vi "GUI_148_AmplifierCams.vi"() -> ()   [LabVIEW 2013]
uses:
  Shared/GUI_Template/GUI_master/tcp_new_data_event.ctl
  Shared/GUI_Template/GUI_master/tcp new data cluster.ctl
  General GUIs/Device GUIs/GUI_Cameras/Controls/Crosshair type def.ctl
  <userlib>/_OpenG.lib/array/array.llb/Filter 1D Array with Scalar (String)__ogtk.vi
panel:
  in  "Analysis::10":bool
  out "MeanCounts::10":dbl caption="updatting?" min=0.0 max=999999999.0 format="%_4g"
  in  "Analysis::9":bool
  out "MeanCounts::9":dbl caption="updatting?" min=0.0 max=999999999.0 format="%_4g"
  in  "Analysis::8":bool
  out "MeanCounts::8":dbl caption="updatting?" min=0.0 max=999999999.0 format="%_4g"
  in  "Analysis::7":bool
  out "MeanCounts::7":dbl caption="updatting?" min=0.0 max=999999999.0 format="%_4g"
  in  "Analysis::6":bool
  out "MeanCounts::6":dbl caption="updatting?" min=0.0 max=999999999.0 format="%_4g"
  in  "Analysis::5":bool
  out "MeanCounts::5":dbl caption="updatting?" min=0.0 max=999999999.0 format="%_4g"
  in  "Analysis::4":bool
  out "MeanCounts::4":dbl caption="updatting?" min=0.0 max=999999999.0 format="%_4g"
  in  "Analysis::3":bool
  out "MeanCounts::3":dbl caption="updatting?" min=0.0 max=999999999.0 format="%_4g"
  in  "Color":u32
  in  "Analysis::2":bool
  out "MeanCounts::2":dbl caption="updatting?" min=0.0 max=999999999.0 format="%_4g"
  in  "triggerdelay::10":dbl=0.001 caption="triggerdelay" min=0.0 max=50000.0 format="%_4p"
  in  "triggerdelay::9":dbl=0.001 caption="triggerdelay" min=0.0 max=0.3 format="%_4p"
  in  "triggerdelay::8":dbl=0.001 caption="triggerdelay" min=16.0 max=50000.0 format="%_4p"
  in  "trigger::10":bool caption="Trigger"
  in  "exposure::10":dbl=0.001 caption="exposure" min=0.0001 max=1.0 format="%_4p"
  in  "trigger::9":bool caption="Trigger"
  in  "exposure::9":dbl=0.001 caption="exposure" min=2e-05 max=1.0 format="%_4p"
  in  "trigger::8":bool caption="Trigger"
  in  "exposure::8":dbl=0.001 caption="exposure" min=0.0001 max=1.0 format="%_4p"
  in  "Target.Y::10":dbl=45.0 caption="y" min=0.0 max=2000.0 format="%#_6f"
  in  "Target.X::10":dbl=47.0 caption="x" min=0.0 max=2000.0 format="%#_6f"
  in  "Target.Y::9":dbl=45.0 caption="y" min=0.0 max=2000.0 format="%#_6f"
  in  "Target.X::9":dbl=47.0 caption="x" min=0.0 max=2000.0 format="%#_6f"
  in  "Target.Y::8":dbl=45.0 caption="y" min=0.0 max=2000.0 format="%#_6f"
  in  "Target.X::8":dbl=47.0 caption="x" min=0.0 max=2000.0 format="%#_6f"
  in  "TargetSize.Y::10":dbl=45.0 caption="y" min=2.0 max=3000.0 format="%#_6f"
  in  "TargetSize.X::10":dbl=47.0 caption="x" min=2.0 max=3000.0 format="%#_6f"
  in  "TargetSize.Y::9":dbl=45.0 caption="y" min=2.0 max=3000.0 format="%#_6f"
  in  "TargetSize.X::9":dbl=47.0 caption="x" min=2.0 max=3000.0 format="%#_6f"
  in  "TargetSize.Y::8":dbl=45.0 caption="y" min=2.0 max=3000.0 format="%#_6f"
  in  "TargetSize.X::8":dbl=47.0 caption="x" min=2.0 max=3000.0 format="%#_6f"
  out "image::10":T1(plugin-control) caption="UC_GAIAMode"
  in  "GUIdevice 10":string="UC_GaiaMode"
  out "image::9":T1(plugin-control) caption="UC_GratingMode"
  in  "GUIdevice 9":string="UC_GratingMode"
  out "image::8":T1(plugin-control) caption="UC_Amp4_IR_output"
  in  "GUIdevice 8":string="UC_Amp4_IR_output"
  in  "TargetSize.Y::7":dbl=45.0 caption="y" min=2.0 max=3000.0 format="%#_6f"
  in  "TargetSize.X::7":dbl=47.0 caption="x" min=2.0 max=3000.0 format="%#_6f"
  in  "TargetSize.Y::6":dbl=45.0 caption="y" min=2.0 max=3000.0 format="%#_6f"
  in  "TargetSize.X::6":dbl=47.0 caption="x" min=2.0 max=3000.0 format="%#_6f"
  in  "TargetSize.Y::5":dbl=45.0 caption="y" min=2.0 max=3000.0 format="%#_6f"
  in  "TargetSize.X::5":dbl=47.0 caption="x" min=2.0 max=3000.0 format="%#_6f"
  in  "TargetSize.Y::4":dbl=45.0 caption="y" min=2.0 max=3000.0 format="%#_6f"
  in  "TargetSize.X::4":dbl=47.0 caption="x" min=2.0 max=3000.0 format="%#_6f"
  in  "TargetSize.Y::3":dbl=163.0 caption="y" min=2.0 max=3000.0 format="%#_6f"
  in  "TargetSize.X::3":dbl=152.0 caption="x" min=2.0 max=3000.0 format="%#_6f"
  in  "TargetSize.Y::2":dbl=74.0 caption="y" min=2.0 max=3000.0 format="%#_6f"
  in  "TargetSize.X::2":dbl=75.0 caption="x" min=2.0 max=3000.0 format="%#_6f"
  in  "active cams":string
  out "CCDs":string[](array[string])
  out "Cameras":T2
  in  "Target.Y::7":dbl=45.0 caption="y" min=0.0 max=2000.0 format="%#_6f"
  in  "Target.X::7":dbl=47.0 caption="x" min=0.0 max=2000.0 format="%#_6f"
  in  "Target.Y::6":dbl=45.0 caption="y" min=0.0 max=2000.0 format="%#_6f"
  in  "Target.X::6":dbl=47.0 caption="x" min=0.0 max=2000.0 format="%#_6f"
  in  "Target.Y::5":dbl=45.0 caption="y" min=0.0 max=2000.0 format="%#_6f"
  in  "Target.X::5":dbl=47.0 caption="x" min=0.0 max=2000.0 format="%#_6f"
  in  "Target.Y::4":dbl=45.0 caption="y" min=0.0 max=2000.0 format="%#_6f"
  in  "Target.X::4":dbl=47.0 caption="x" min=0.0 max=2000.0 format="%#_6f"
  in  "Target.Y::3":dbl=163.0 caption="y" min=0.0 max=2000.0 format="%#_6f"
  in  "Target.X::3":dbl=152.0 caption="x" min=0.0 max=2000.0 format="%#_6f"
  in  "Target.Y::2":dbl=74.0 caption="y" min=0.0 max=2000.0 format="%#_6f"
  in  "Target.X::2":dbl=75.0 caption="x" min=0.0 max=2000.0 format="%#_6f"
  out "error out":errorcluster
  out "image::7":T1(plugin-control) caption="UC_Amp4Depletion_South"
  in  "triggerdelay::7":dbl=0.001 caption="triggerdelay" min=10.0 max=50000.0 format="%_4p"
  in  "triggerdelay::6":dbl=0.001 caption="triggerdelay" min=20.0 max=50000.0 format="%_4p"
  in  "triggerdelay::5":dbl=0.001 caption="triggerdelay" min=10.0 max=50000.0 format="%_4p"
  in  "triggerdelay::4":dbl=0.001 caption="triggerdelay" min=20.0 max=50000.0 format="%_4p"
  in  "triggerdelay::3":dbl=0.001 caption="triggerdelay" min=20.0 max=50000.0 format="%_4p"
  in  "triggerdelay::2":dbl=0.001 caption="triggerdelay" min=0.0 max=50000.0 format="%_4p"
  in  "trigger::7":bool caption="Trigger"
  in  "exposure::7":dbl=0.001 caption="exposure" min=0.0001 max=1.0 format="%_4p"
  in  "GUIdevice 7":string="UC_Amp4Depletion_South"
  in  "trigger::6":bool caption="Trigger"
  in  "exposure::6":dbl=0.001 caption="exposure" min=0.0001 max=1.0 format="%_4p"
  out "image::6":T1(plugin-control) caption="UC_Amp3Depletion_South"
  in  "GUIdevice 6":string="UC_Amp3Depletion_South"
  in  "trigger::5":bool caption="Trigger"
  in  "exposure::5":dbl=0.001 caption="exposure" min=0.0001 max=1.0 format="%_4p"
  out "image::5":T1(plugin-control) caption="UC_Amp2Depletion_South"
  in  "GUIdevice 5":string="UC_Amp2Depletion_South"
  in  "trigger::4":bool caption="Trigger"
  in  "exposure::4":dbl=0.001 caption="exposure" min=0.0001 max=1.0 format="%_4p"
  out "image::4":T1(plugin-control) caption="UC_Amp4_IR_Input"
  in  "GUIdevice 4":string="UC_Amp4_IR_input"
  in  "trigger::3":bool caption="Trigger"
  in  "exposure::3":dbl=0.001 caption="exposure" min=0.0001 max=1.0 format="%_4p"
  out "image::3":T1(plugin-control) caption="UC_Amp3_IR_Input"
  in  "GUIdevice 3":string="UC_Amp3_IR_input"
  in  "trigger::2":bool caption="Trigger"
  in  "exposure::2":dbl=0.001 caption="exposure" min=0.0001 max=1.0 format="%_4p"
  out "image::2":T1(plugin-control) caption="UC_Amp2_IR_input"
  in  "GUIdevice 2":string="UC_Amp2_IR_input"
  out "tcp data event":T3
  in  "Select device":string(combo)="FrogHPD"
  in  "stop":bool
  in  "GUIdevice 1":string="HPD_CCD"
  # "XHair location"
  # "XHair size"
  # "XHair location"
  # "XHair size"
  # "XHair location"
  # "XHair size"
  # "XHair location"
  # "XHair size"
  # "XHair location"
  # "XHair size"
  # "XHair location"
  # "XHair size"
  # "XHair location"
  # "XHair size"
  # "XHair location"
  # "XHair size"
  # "XHair location"
  # "XHair size"
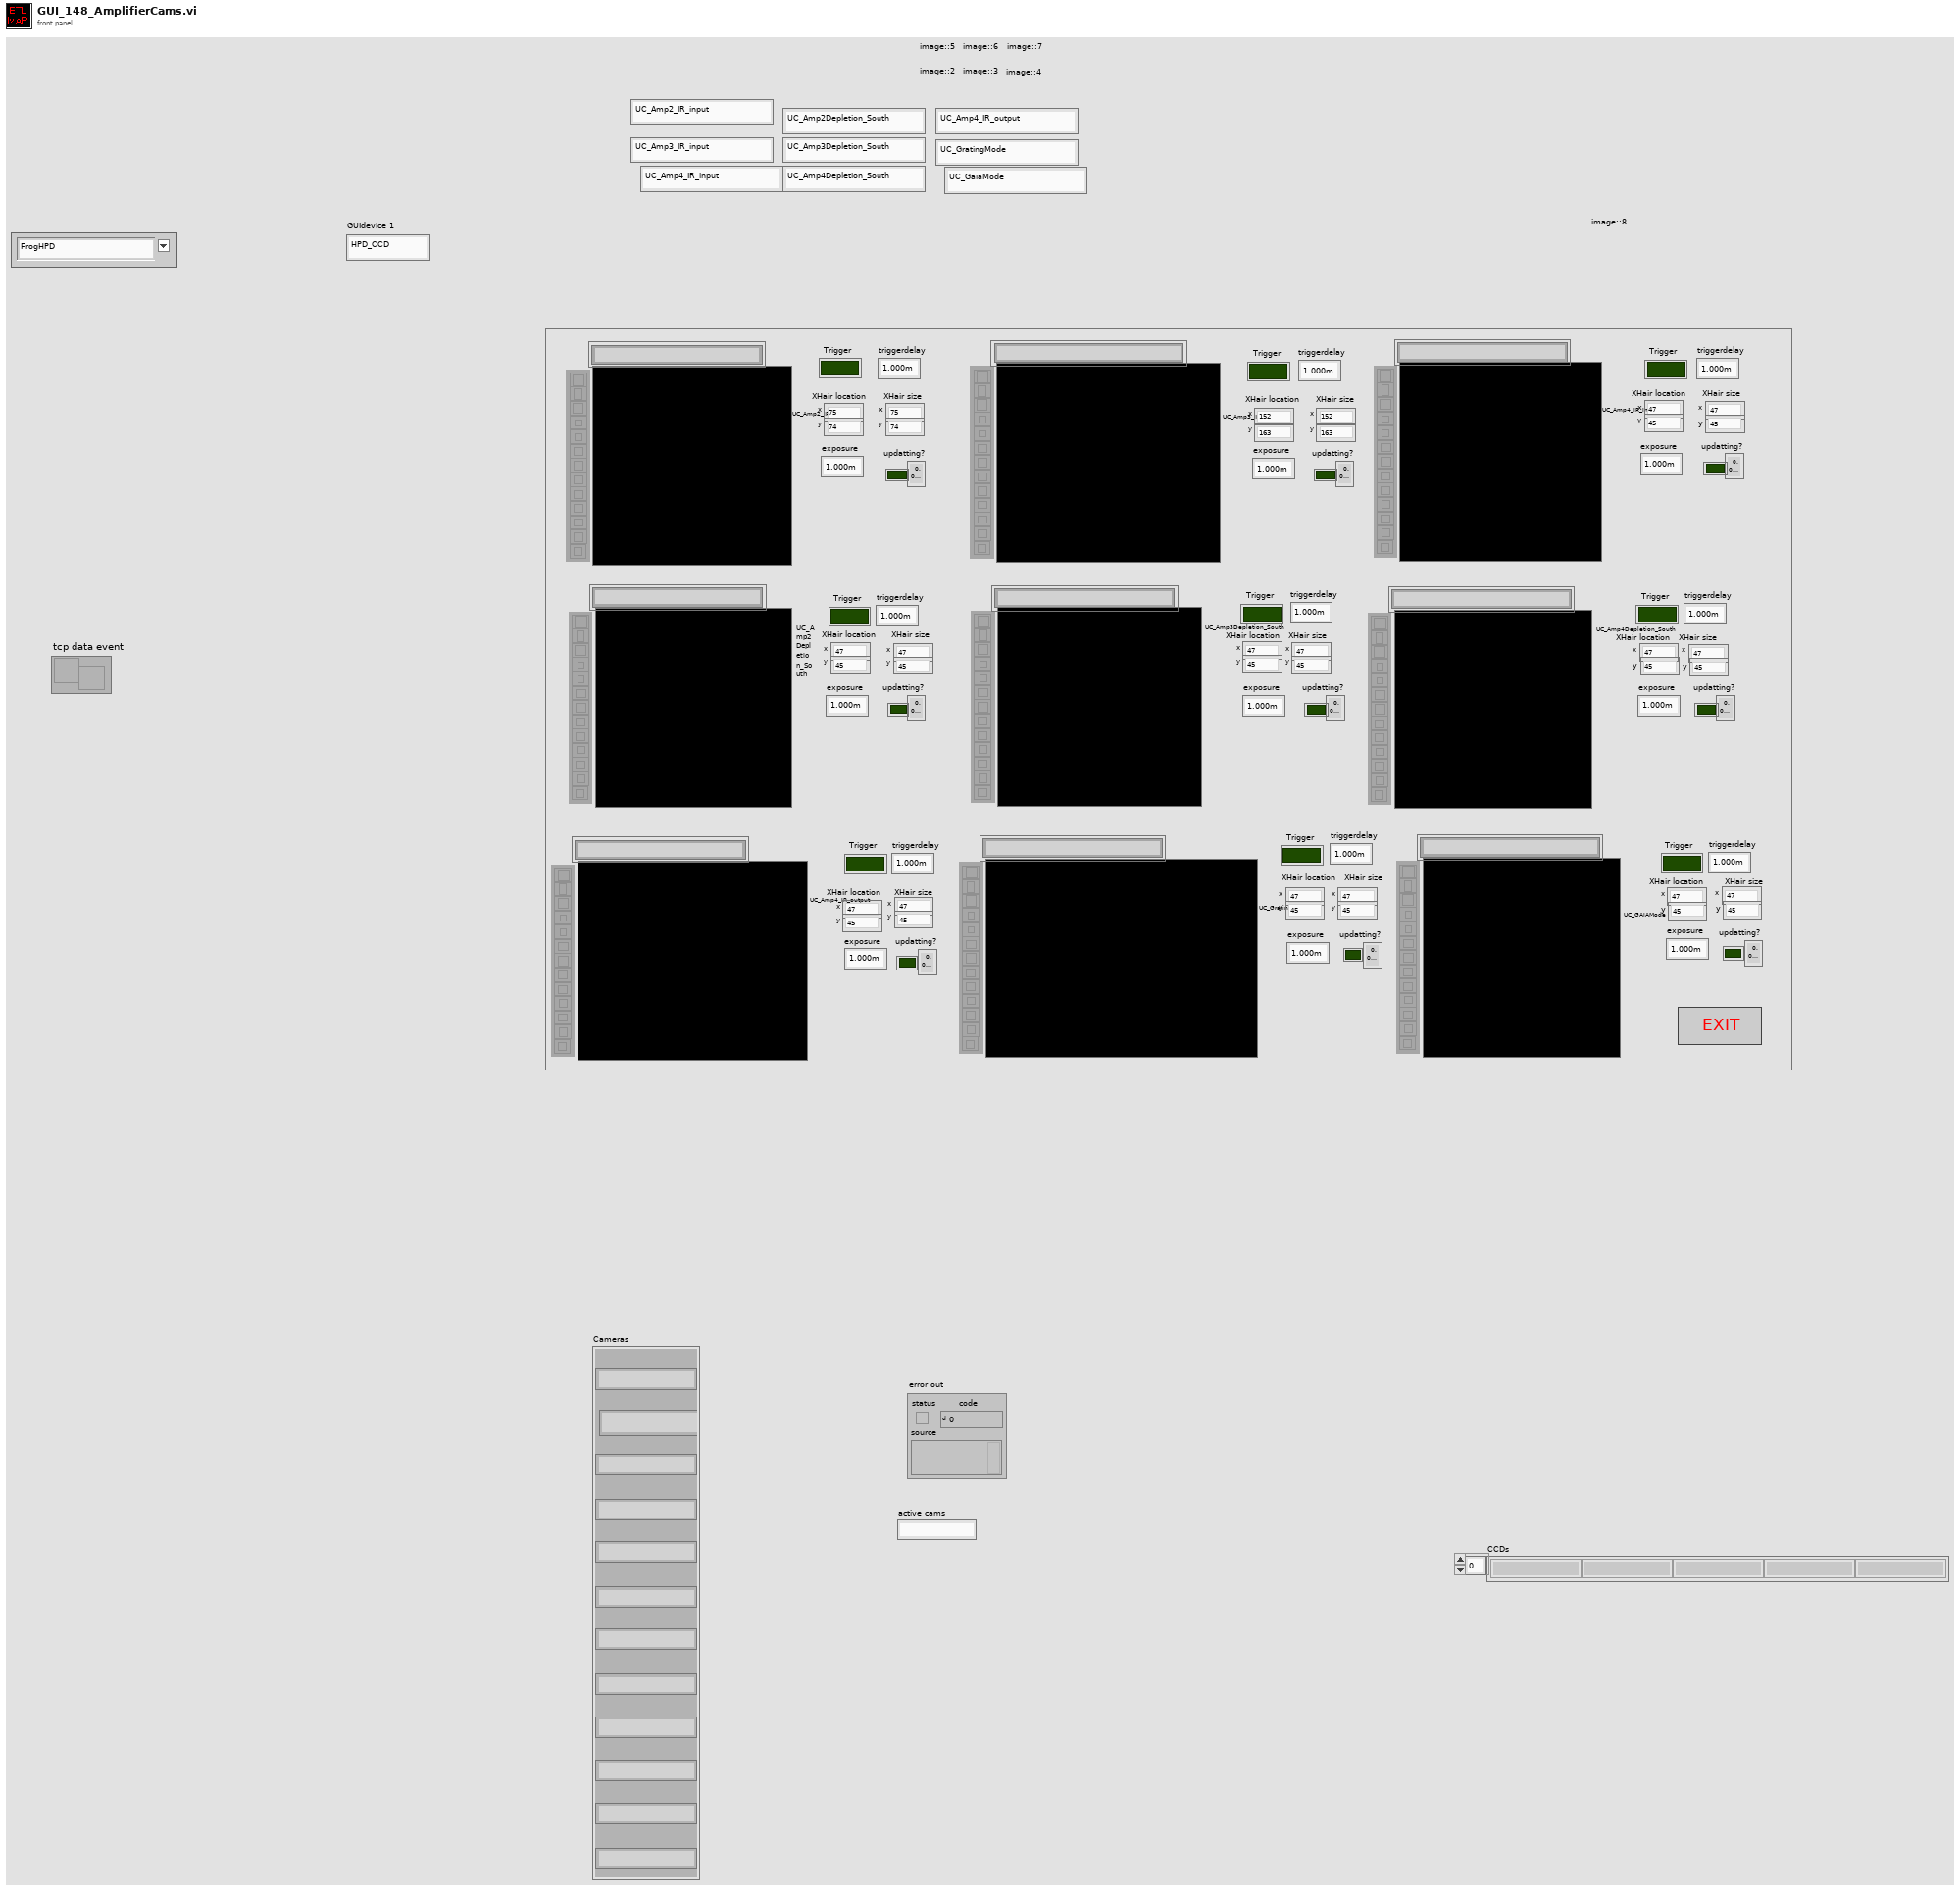
[diagram p1: front panel]
types:
  T1 = typedef "IMAQ Image.ctl" = refnum<image>
  T2 = cluster{"[0]":string, "[1]":string, "[2]":string, "[3]":string, "[4]":string, "[5]":string, "[6]":string, "[7]":string, "[8]":string, "[8] 2":string, "[8] 3":string, "[8] 4":string}
  T3 = typedef "tcp_new_data_event.ctl" = refnum<user-event>
  T4 = typedef "Image Type" = u32
  T5 = cluster{"Target.X::8":refnum<vi>, "Target.Y::8":refnum<vi>}
  T6 = cluster{"Target.X::9":refnum<vi>, "Target.Y::9":refnum<vi>}
  T7 = cluster{"Target.X::10":refnum<vi>, "Target.Y::10":refnum<vi>}
  T8 = cluster{"Target.X::2":refnum<vi>, "Target.Y::2":refnum<vi>}
  T9 = cluster{"Target.X::3":refnum<vi>, "Target.Y::3":refnum<vi>}
  T10 = cluster{"Target.X::4":refnum<vi>, "Target.Y::4":refnum<vi>}
  T11 = cluster{"Target.X::5":refnum<vi>, "Target.Y::5":refnum<vi>}
  T12 = cluster{"Target.X::6":refnum<vi>, "Target.Y::6":refnum<vi>}
  T13 = cluster{"Target.X::7":refnum<vi>, "Target.Y::7":refnum<vi>}
  T14 = cluster{"TargetSize.X::4":refnum<vi>, "TargetSize.Y::4":refnum<vi>}
  T15 = cluster{"TargetSize.X::5":refnum<vi>, "TargetSize.Y::5":refnum<vi>}
  T16 = cluster{"TargetSize.X::6":refnum<vi>, "TargetSize.Y::6":refnum<vi>}
  T17 = cluster{"TargetSize.X::7":refnum<vi>, "TargetSize.Y::7":refnum<vi>}
  T18 = cluster{"TargetSize.X::8":refnum<vi>, "TargetSize.Y::8":refnum<vi>}
  T19 = cluster{"TargetSize.X::9":refnum<vi>, "TargetSize.Y::9":refnum<vi>}
  T20 = cluster{"TargetSize.X::10":refnum<vi>, "TargetSize.Y::10":refnum<vi>}
  T21 = cluster{"TargetSize.X::2":refnum<vi>, "TargetSize.Y::2":refnum<vi>}
  T22 = cluster{"TargetSize.X::3":refnum<vi>, "TargetSize.Y::3":refnum<vi>}
  T23 = cluster{"[0]":string, "[1]":string, "[2]":string, "[3]":string, "[4]":string, "[5]":string, "[6]":string, "[7]":string, "[8]":string, "[9]":string, "[10]":string, "[11]":string}
  T24 = cluster{"TargetSize.X::10":refnum<vi>, "TargetSize.Y::10":refnum<vi>}[]
  T25 = cluster{"Target.X::10":refnum<vi>, "Target.Y::10":refnum<vi>}[]
  T26 = typedef "Crosshair type def.ctl" = cluster{"Draw":bool, "Target":cluster{"x":dbl, "y":dbl}, "Size":cluster{"x":dbl, "y":dbl}, "Angle":dbl, "Color":u32, "Thickness":u8, "CrosshairLabel":string}
  T27 = cluster{"Left":i32, "Top":i32, "Right":i32, "Bottom":i32}
  T28 = enum32{"invalid app kind", "Development System", "Run Time System", "Student Edition", "Embedded LabVIEW", "Evaluation", "Custom"}
  T29 = typedef "tcp new data cluster.ctl" = cluster{"EventEnum":enum16{"new data", "connection status update"}, "Device name":string}
  T30 = enum32{"Invalid", "Standard", "Closed", "Hidden", "Minimized", "Maximized"}
  T31 = cluster{"Core":cluster{"Current VI Reference":refnum<vi>, "Close Panel on Exit?":bool}, "Your Boolean data":bool, "active cams":string, "SuperGUI":cluster{"STOP queue":refnum<queue>, "SuperGUI ref":refnum<vi>}}
  T32 = cluster{"STOP queue":refnum<queue>, "SuperGUI ref":refnum<vi>}
  T33 = cluster{"Current VI Reference":refnum<vi>, "Close Panel on Exit?":bool}
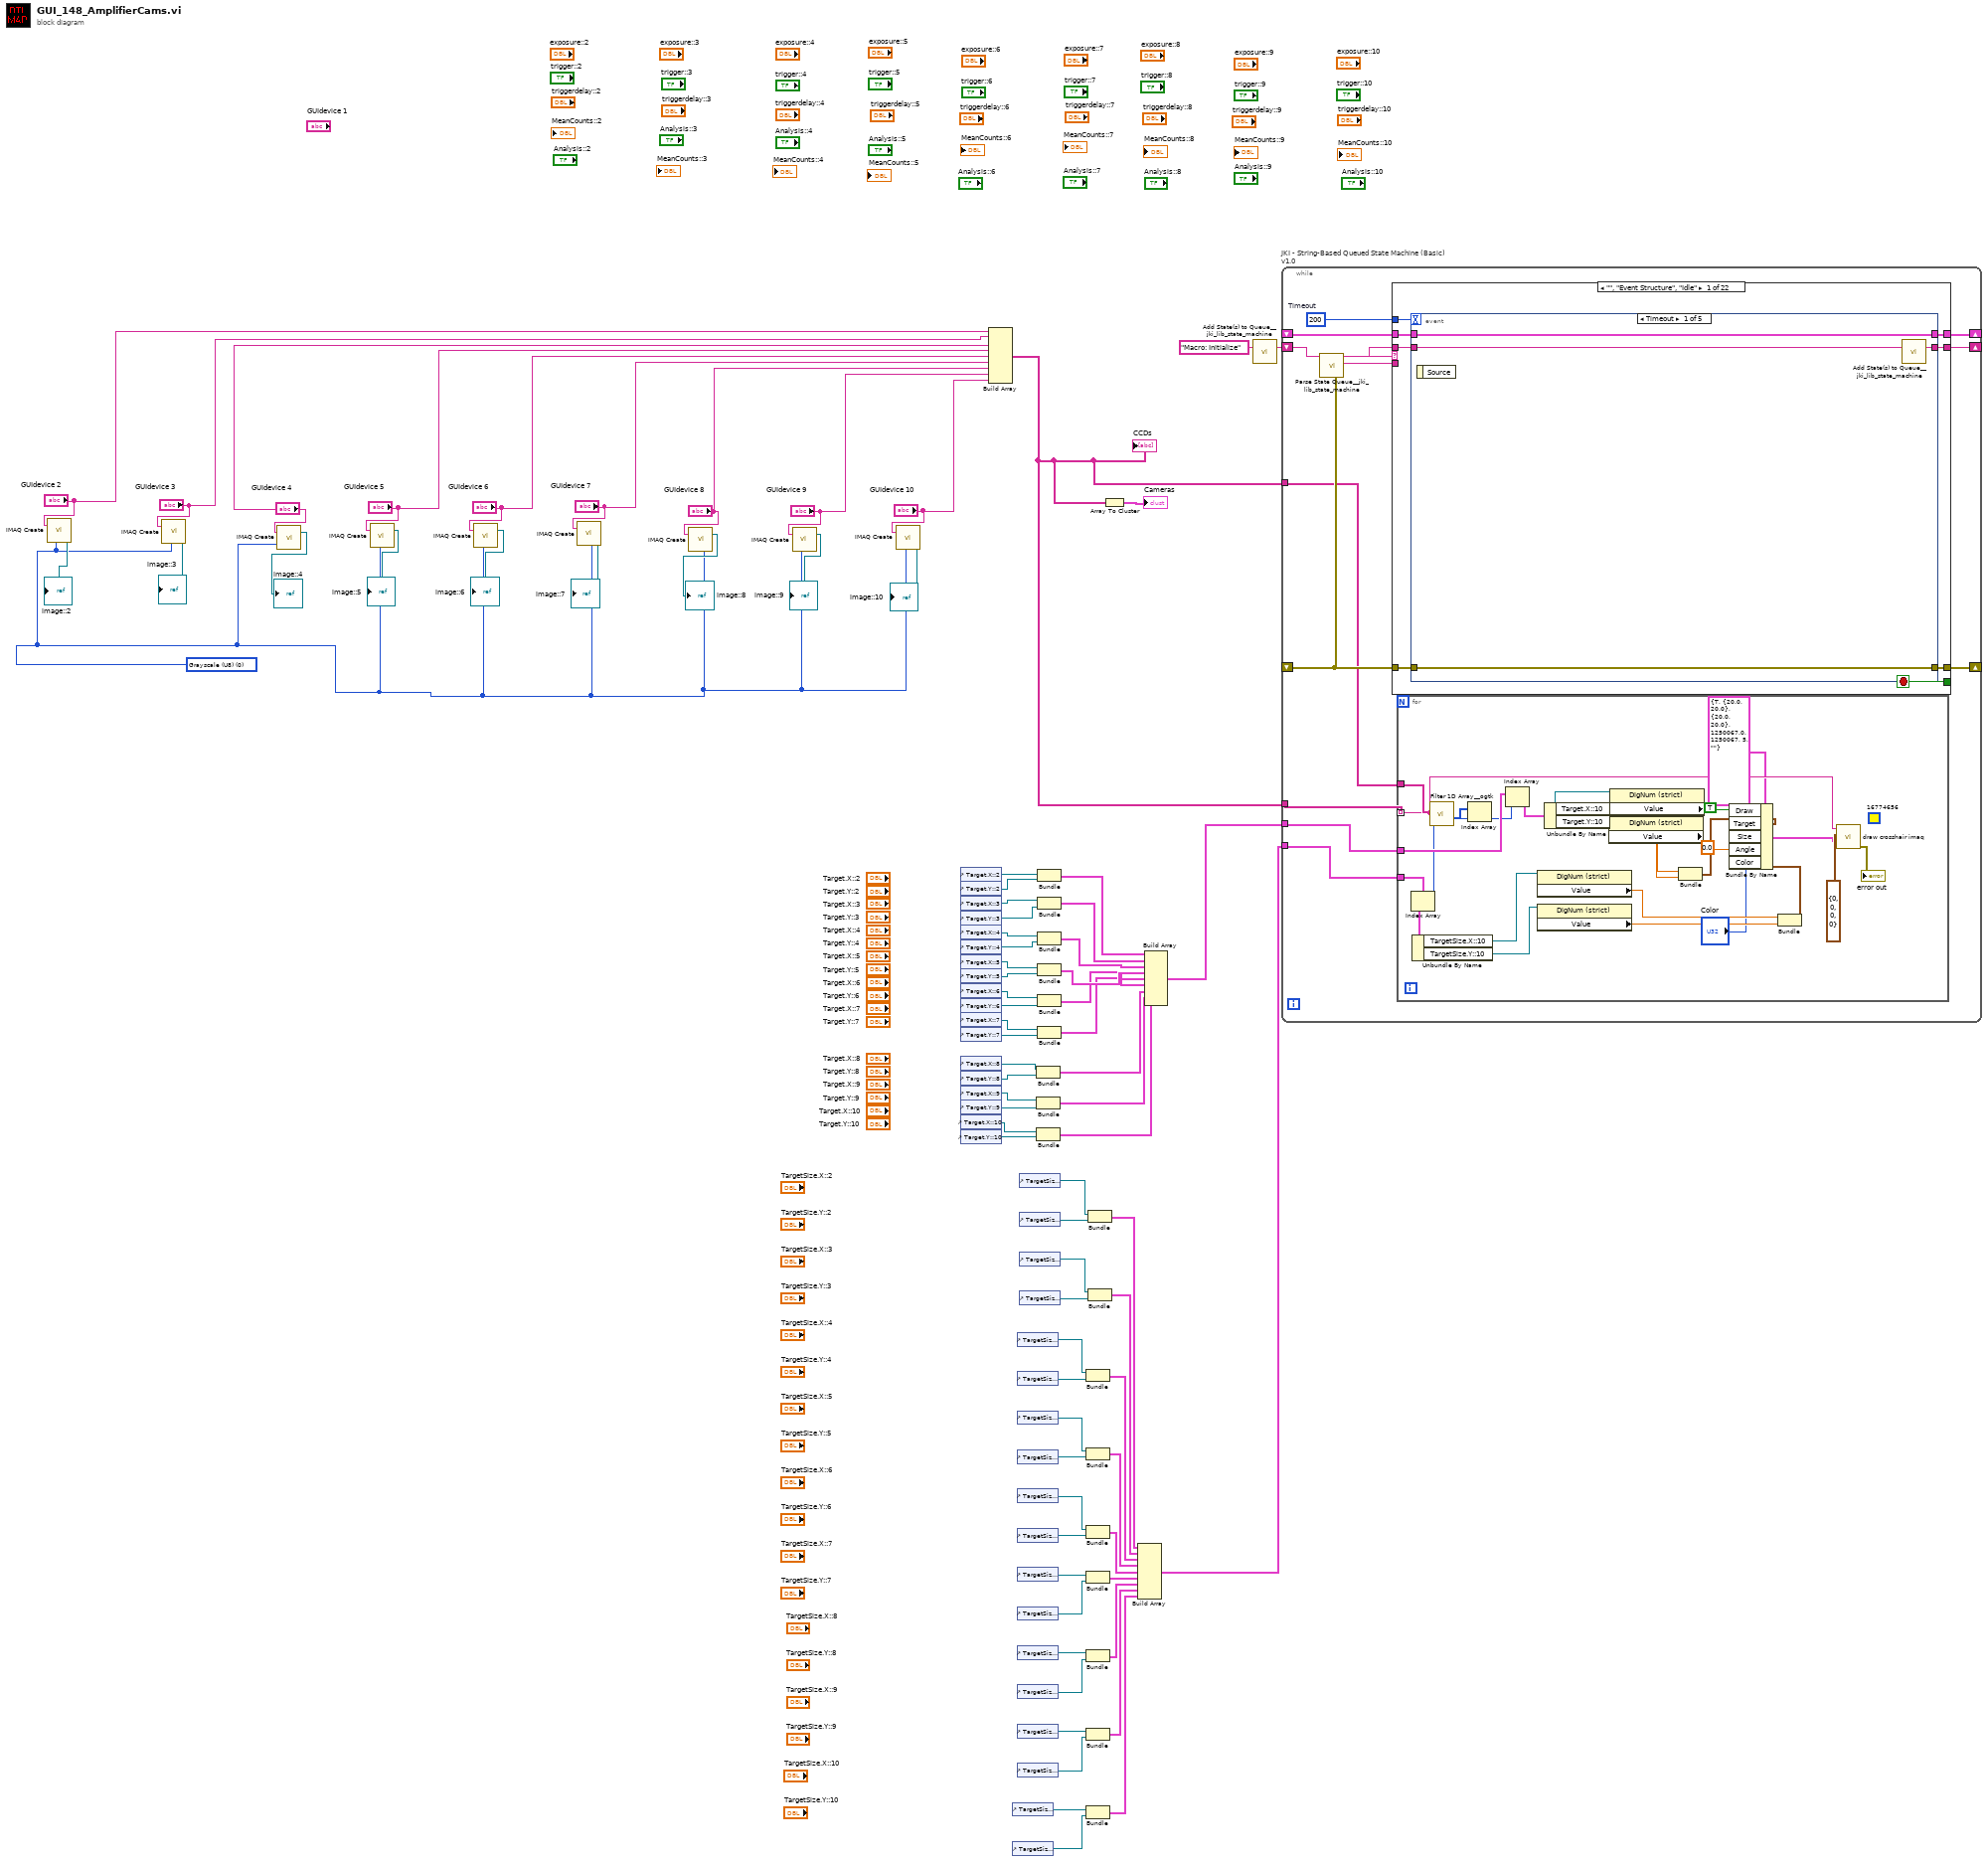
[diagram p0: block diagram]
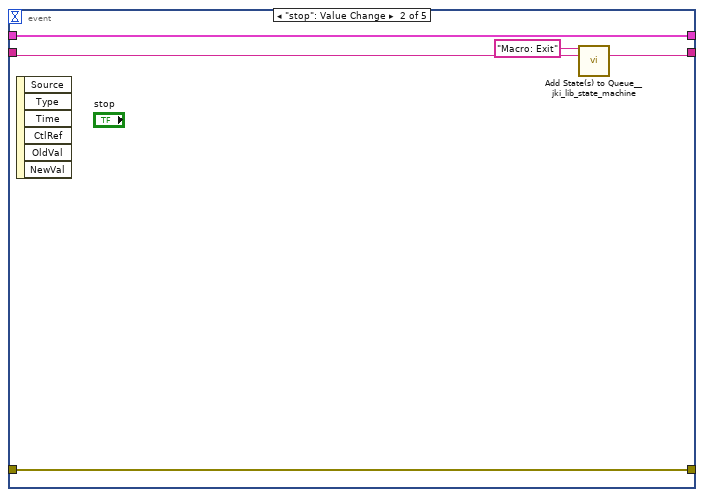
[diagram p2: hidden frame]
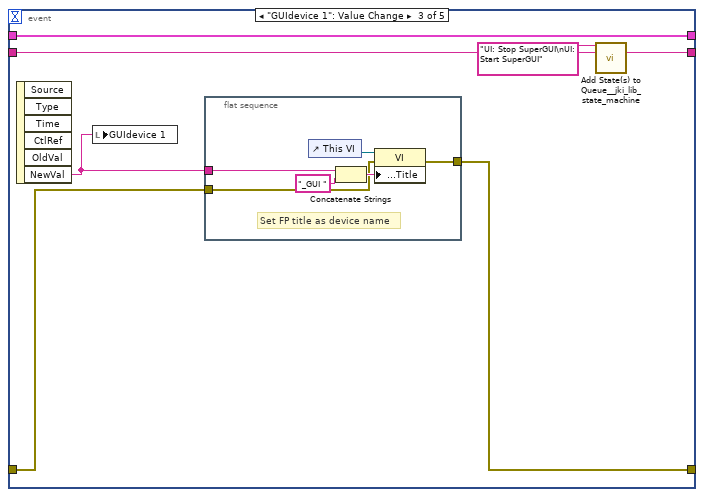
[diagram p3: hidden frame]
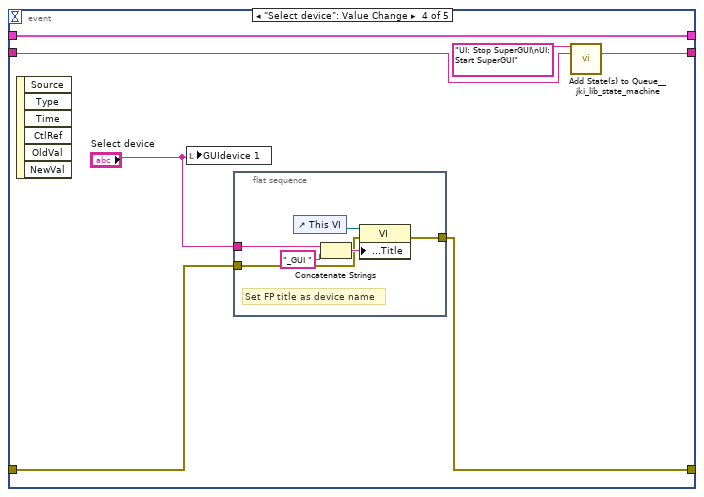
[diagram p4: hidden frame]
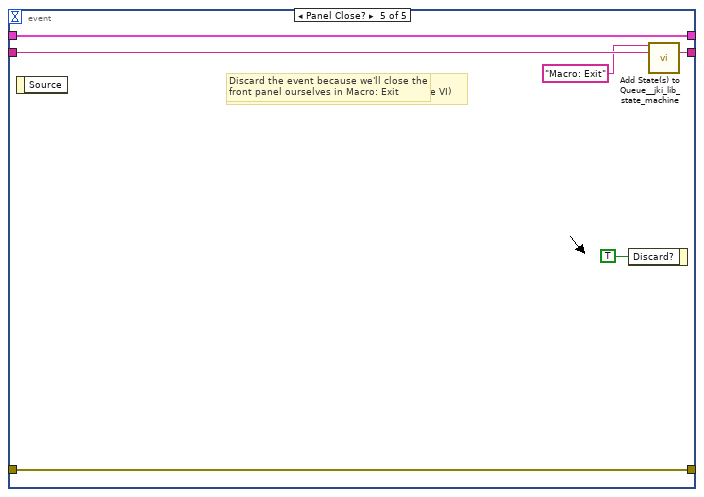
[diagram p5: hidden frame]
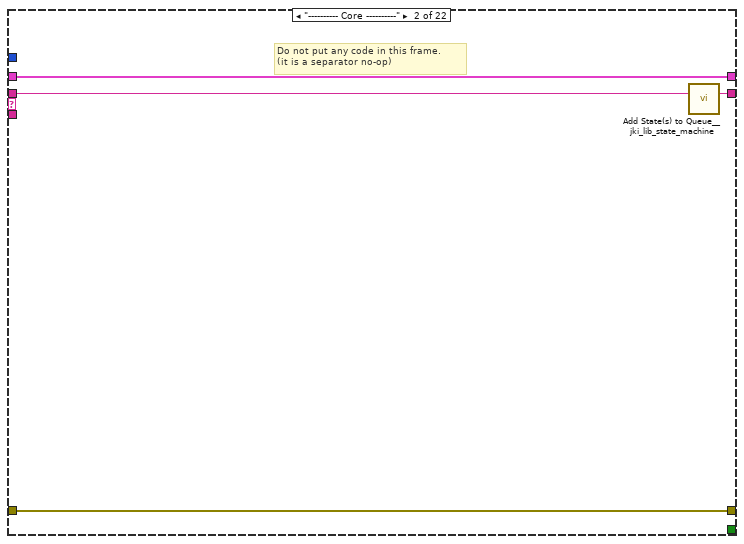
[diagram p6: hidden frame]
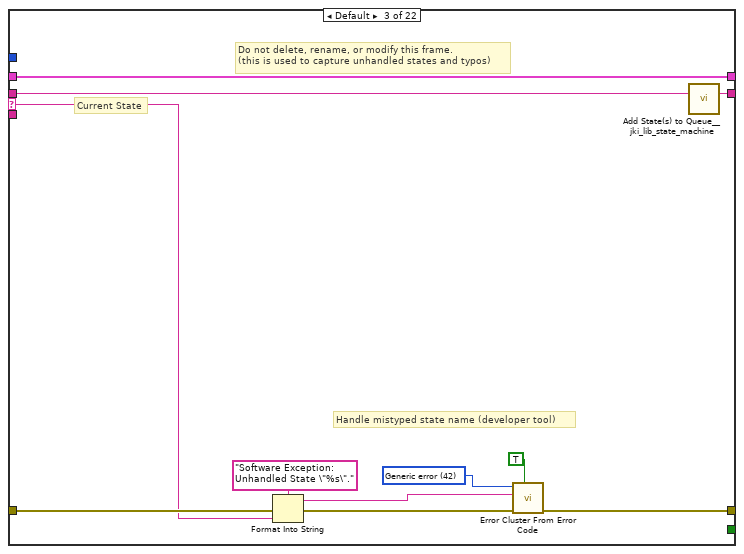
[diagram p7: hidden frame]
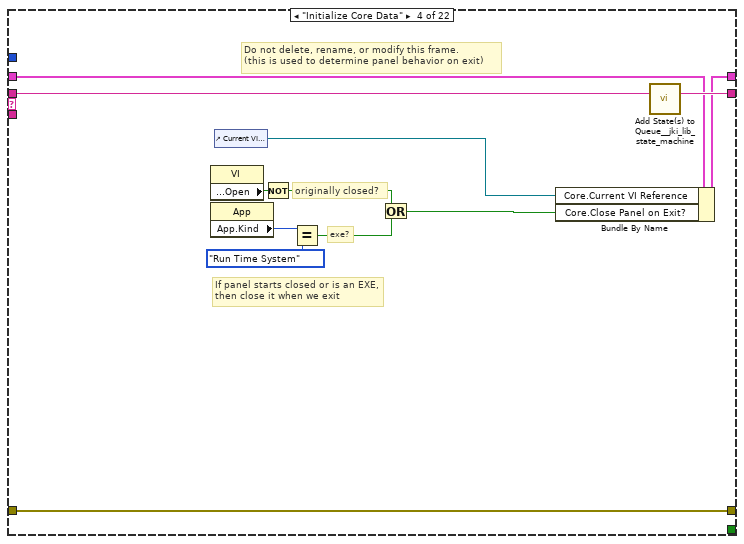
[diagram p8: hidden frame]
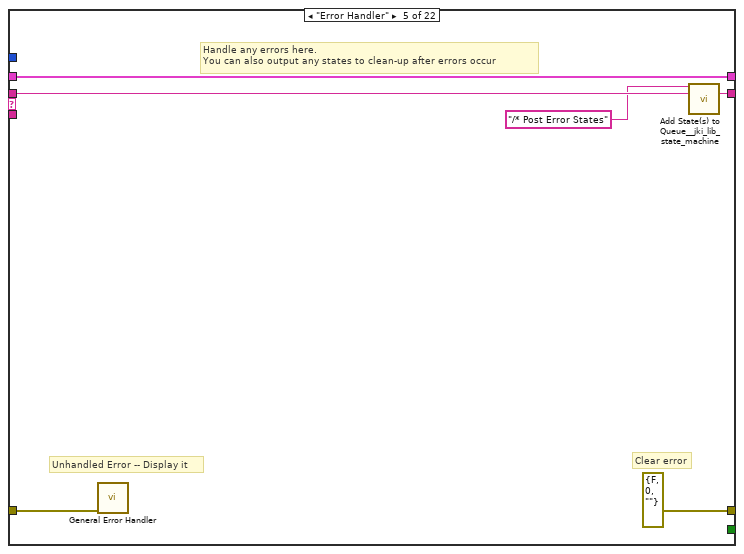
[diagram p9: hidden frame]
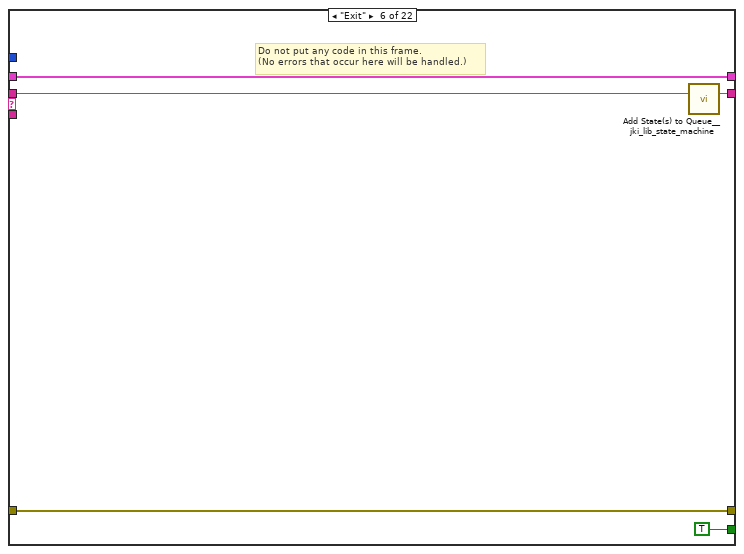
[diagram p10: hidden frame]
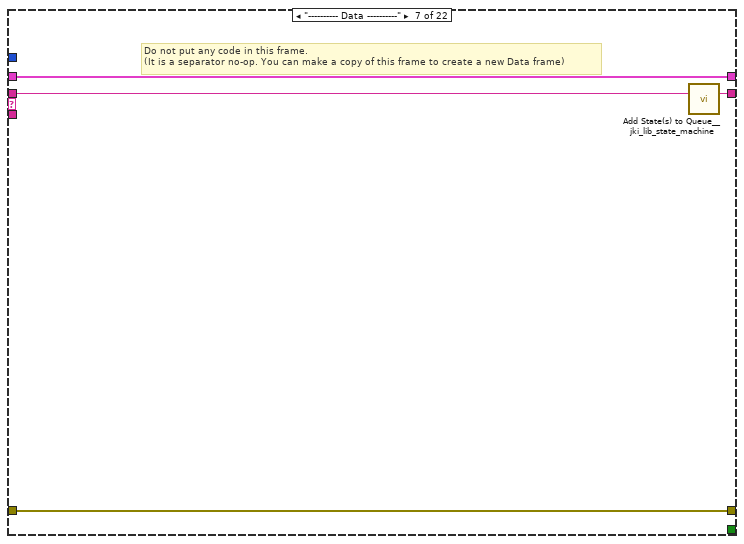
[diagram p11: hidden frame]
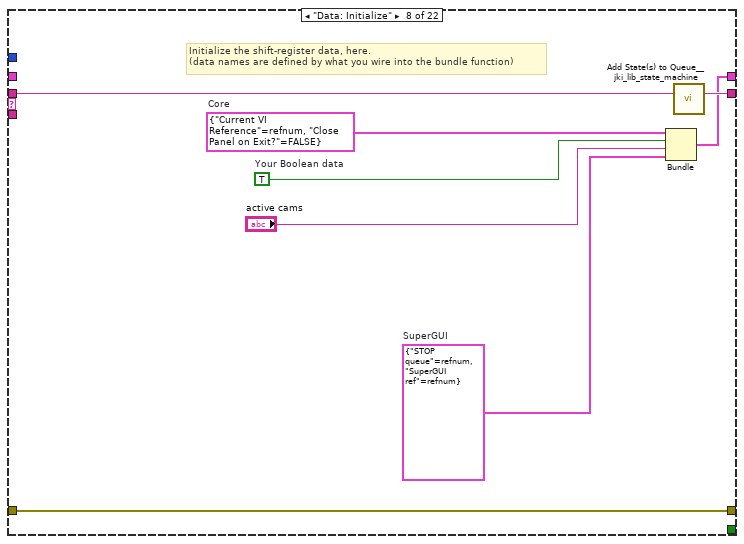
[diagram p12: hidden frame]
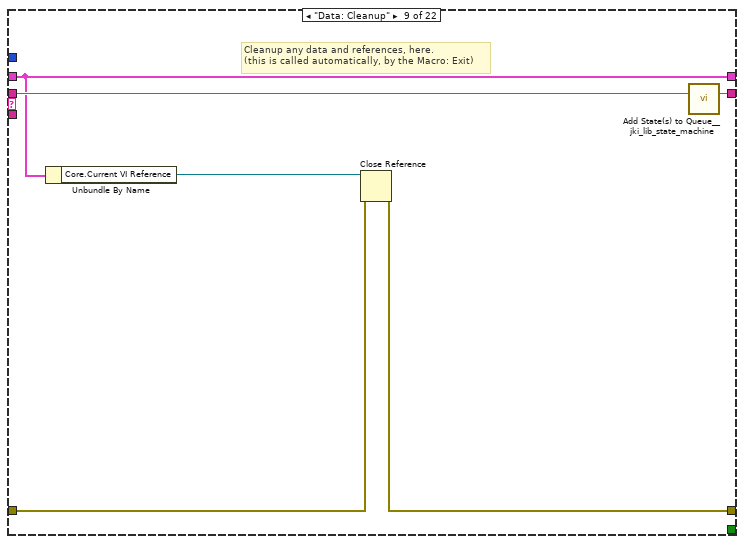
[diagram p13: hidden frame]
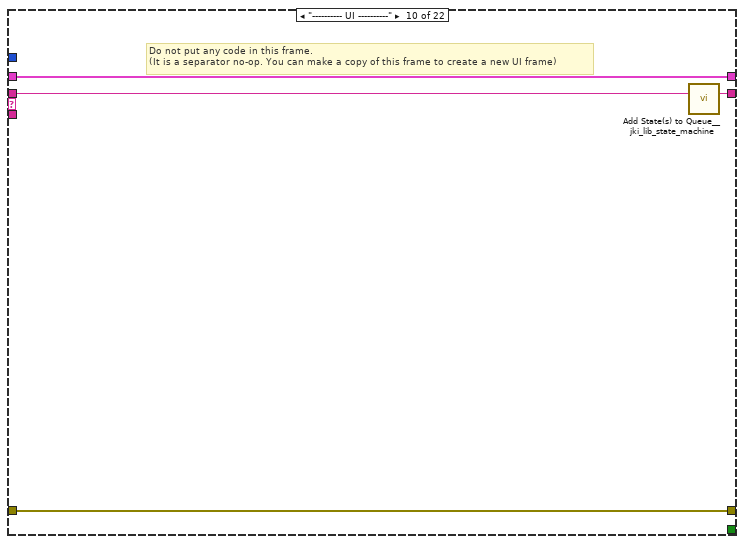
[diagram p14: hidden frame]
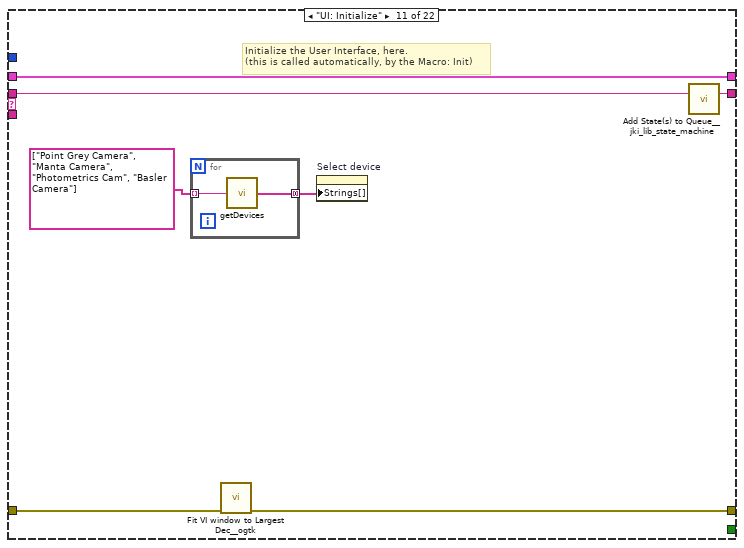
[diagram p15: hidden frame]
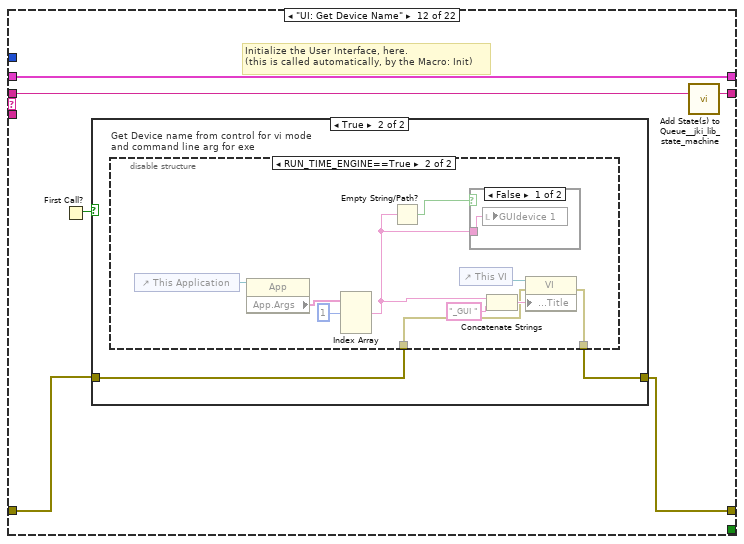
[diagram p16: hidden frame]
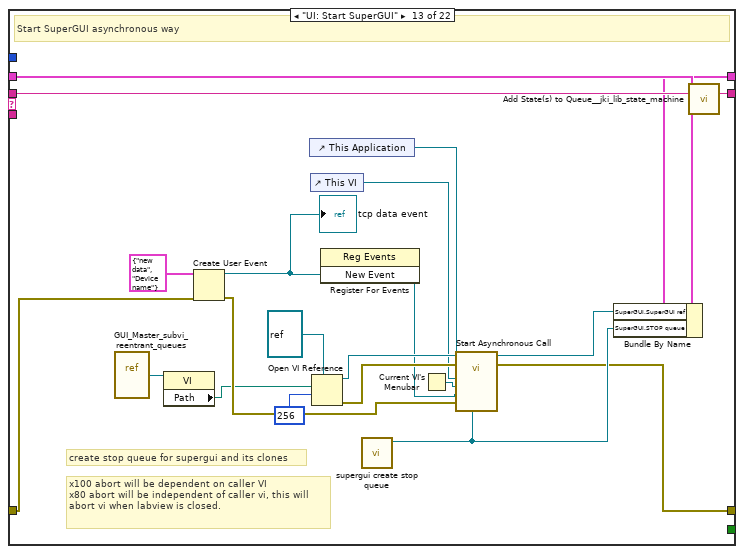
[diagram p20: hidden frame]
diagram:
  w22 = T4 0 items=["Grayscale (U8)", "Grayscale (I16)", "Grayscale (SGL)", "Complex (CSG)", "RGB (U32)", "HSL (U32)", "RGB (U64)", "Grayscale (U16)"] ("Image Type")
  n1 = call "IMAQ Create"("Image Name"="GUIdevice 2", "Image Type"=w22) -> ("New Image"=→"image::2":T1)  [unwired: 3 in, 1 out]
  n2 = call "IMAQ Create"("Image Name"="GUIdevice 3", "Image Type"=w22) -> ("New Image"=→"image::3":T1)  [unwired: 3 in, 1 out]
  n3 = call "IMAQ Create"("Image Name"="GUIdevice 4", "Image Type"=w22) -> ("New Image"=→"image::4":T1)  [unwired: 3 in, 1 out]
  n4 = call "IMAQ Create"("Image Name"="GUIdevice 5", "Image Type"=w22) -> ("New Image"=→"image::5":T1)  [unwired: 3 in, 1 out]
  n5 = call "IMAQ Create"("Image Name"="GUIdevice 6", "Image Type"=w22) -> ("New Image"=→"image::6":T1)  [unwired: 3 in, 1 out]
  n6 = call "IMAQ Create"("Image Name"="GUIdevice 7", "Image Type"=w22) -> ("New Image"=→"image::7":T1)  [unwired: 3 in, 1 out]
  n7 = call "IMAQ Create"("Image Name"="GUIdevice 8", "Image Type"=w22) -> ("New Image"=→"image::8":T1)  [unwired: 3 in, 1 out]
  n8 = call "IMAQ Create"("Image Name"="GUIdevice 9", "Image Type"=w22) -> ("New Image"=→"image::9":T1)  [unwired: 3 in, 1 out]
  n9 = call "IMAQ Create"("Image Name"="GUIdevice 10", "Image Type"=w22) -> ("New Image"=→"image::10":T1)  [unwired: 3 in, 1 out]
  n10 = control-ref of="Target.X::2"() -> (w71:refnum<vi>)
  n11 = control-ref of="Target.Y::2"() -> (w70:refnum<vi>)
  n12 = control-ref of="Target.X::3"() -> (w69:refnum<vi>)
  n13 = control-ref of="Target.Y::3"() -> (w68:refnum<vi>)
  n14 = control-ref of="Target.X::4"() -> (w67:refnum<vi>)
  n15 = control-ref of="Target.Y::4"() -> (w66:refnum<vi>)
  n16 = control-ref of="Target.X::5"() -> (w65:refnum<vi>)
  n17 = control-ref of="Target.Y::5"() -> (w64:refnum<vi>)
  n18 = control-ref of="Target.X::6"() -> (w63:refnum<vi>)
  n19 = control-ref of="Target.Y::6"() -> (w62:refnum<vi>)
  n20 = control-ref of="Target.X::7"() -> (w61:refnum<vi>)
  n21 = control-ref of="Target.Y::7"() -> (w60:refnum<vi>)
  n22 = control-ref of="Target.X::8"() -> (w6:refnum<vi>)
  n23 = control-ref of="Target.Y::8"() -> (w5:refnum<vi>)
  n24 = control-ref of="Target.X::9"() -> (w4:refnum<vi>)
  n25 = control-ref of="Target.Y::9"() -> (w3:refnum<vi>)
  n26 = control-ref of="Target.X::10"() -> (w2:refnum<vi>)
  n27 = control-ref of="Target.Y::10"() -> (w1:refnum<vi>)
  n28 = Build Array("GUIdevice 2", "GUIdevice 3", "GUIdevice 4", "GUIdevice 5", "GUIdevice 6", "GUIdevice 7", "GUIdevice 8", "GUIdevice 9", "GUIdevice 10") -> (w45:string[])
  "CCDs" <- w45
  n29 = control-ref of="TargetSize.X::10"() -> (w11:refnum<vi>)
  n30 = control-ref of="TargetSize.Y::10"() -> (w10:refnum<vi>)
  n31 = control-ref of="TargetSize.X::4"() -> (w40:refnum<vi>)
  n32 = control-ref of="TargetSize.Y::4"() -> (w39:refnum<vi>)
  n33 = control-ref of="TargetSize.X::5"() -> (w38:refnum<vi>)
  n34 = control-ref of="TargetSize.Y::5"() -> (w37:refnum<vi>)
  n35 = control-ref of="TargetSize.X::6"() -> (w36:refnum<vi>)
  n36 = control-ref of="TargetSize.Y::6"() -> (w35:refnum<vi>)
  n37 = control-ref of="TargetSize.X::7"() -> (w34:refnum<vi>)
  n38 = control-ref of="TargetSize.Y::7"() -> (w33:refnum<vi>)
  n39 = control-ref of="TargetSize.X::8"() -> (w15:refnum<vi>)
  n40 = control-ref of="TargetSize.Y::8"() -> (w14:refnum<vi>)
  n41 = control-ref of="TargetSize.X::9"() -> (w13:refnum<vi>)
  n42 = control-ref of="TargetSize.Y::9"() -> (w12:refnum<vi>)
  n43 = control-ref of="TargetSize.X::2"() -> (w44:refnum<vi>)
  n44 = control-ref of="TargetSize.Y::2"() -> (w43:refnum<vi>)
  n45 = control-ref of="TargetSize.X::3"() -> (w42:refnum<vi>)
  n46 = control-ref of="TargetSize.Y::3"() -> (w41:refnum<vi>)
  n47 = Bundle("Target.X::8"=w6, "Target.Y::8"=w5) -> (w18:T5)  [unwired: 1 in]
  n48 = Bundle("Target.X::9"=w4, "Target.Y::9"=w3) -> (w17:T6)  [unwired: 1 in]
  n49 = Bundle("Target.X::10"=w2, "Target.Y::10"=w1) -> (w16:T7)  [unwired: 1 in]
  n50 = Bundle("Target.X::2"=w71, "Target.Y::2"=w70) -> (w59:T8)  [unwired: 1 in]
  n51 = Bundle("Target.X::3"=w69, "Target.Y::3"=w68) -> (w58:T9)  [unwired: 1 in]
  n52 = Bundle("Target.X::4"=w67, "Target.Y::4"=w66) -> (w54:T10)  [unwired: 1 in]
  n53 = Bundle("Target.X::5"=w65, "Target.Y::5"=w64) -> (w57:T11)  [unwired: 1 in]
  n54 = Bundle("Target.X::6"=w63, "Target.Y::6"=w62) -> (w56:T12)  [unwired: 1 in]
  n55 = Bundle("Target.X::7"=w61, "Target.Y::7"=w60) -> (w55:T13)  [unwired: 1 in]
  n56 = Bundle("TargetSize.X::4"=w40, "TargetSize.Y::4"=w39) -> (w27:T14)  [unwired: 1 in]
  n57 = Bundle("TargetSize.X::5"=w38, "TargetSize.Y::5"=w37) -> (w30:T15)  [unwired: 1 in]
  n58 = Bundle("TargetSize.X::6"=w36, "TargetSize.Y::6"=w35) -> (w29:T16)  [unwired: 1 in]
  n59 = Bundle("TargetSize.X::7"=w34, "TargetSize.Y::7"=w33) -> (w28:T17)  [unwired: 1 in]
  n60 = Bundle("TargetSize.X::8"=w15, "TargetSize.Y::8"=w14) -> (w9:T18)  [unwired: 1 in]
  n61 = Bundle("TargetSize.X::9"=w13, "TargetSize.Y::9"=w12) -> (w8:T19)  [unwired: 1 in]
  n62 = Bundle("TargetSize.X::10"=w11, "TargetSize.Y::10"=w10) -> (w7:T20)  [unwired: 1 in]
  n63 = Bundle("TargetSize.X::2"=w44, "TargetSize.Y::2"=w43) -> (w32:T21)  [unwired: 1 in]
  n64 = Bundle("TargetSize.X::3"=w42, "TargetSize.Y::3"=w41) -> (w31:T22)  [unwired: 1 in]
  n65 = Array To Cluster(array=w45) -> (cluster=→"Cameras":T23)
  n66 = Build Array(w32, w31, w27, w30, w29, w28, w9, w8, w7) -> (w26:T24)
  n67 = Build Array(w59, w58, w54, w57, w56, w55, w18, w17, w16) -> (w53:T25)
  n68 = call <vilib>:"Add State(s) to Queue__jki_lib_state_machine.vi"("State(s) in (\"\")"="Macro: Initialize") -> ("States Out"=w79:string)  [unwired: 14 in]
  n69 = while "JKI - String-Based Queued State Machine (Basic) v1.0" {
    shift-right: [w87] -> _
    shift-left: _ -> [w82]
    shift-right: [w90] -> _
    shift-left: _ -> [w85]
    shift-right: [w89] -> _
    shift-left: w79 -> [w91]
    tunnel: w53 -> [w84]
    tunnel: w45 -> [w83]
    tunnel: w45 -> [w81]
    tunnel: w26 -> [w80]
    stop <- w88 stop-if-true
    w86 = 200  # Timeout
    n70 = call <vilib>:"Parse State Queue__jki_lib_state_machine.vi"("State Queue"=w91, "Error In (no error)"=w85) -> ("Remaining States"=w93:string, "Current State"=w94:string, "Arguments"=w92:string)  [unwired: 11 in]
    n71 = case shown="\"\", \"Event Structure\", \"Idle\"" w94 {
      selector: w94 -> [_ _ w172 _ _ _ _ _ _ _ _ _ _ _ _ _ _ _ _ _ _ _]
      tunnel: w93 -> [w126 w171 w176 w194 w200 w205 w209 w217 w223 w227 w234 w242 w277 w285 w291 w302 w328 w333 w343 w347 w351 w355]
      tunnel: w92 -> [_ _ _ _ _ _ _ _ _ _ _ _ _ _ w286 w296 _ _ _ _ _ _]
      tunnel: w82 -> [w124 w168 w174 w185 w197 w203 w206 _ w218 w224 w232 w240 w268 w280 w289 w298 w325 w330 w340 w344 w348 w352]
      tunnel: [w123 w169 w178 w191 errorcluster {"status"=FALSE, "code"=0, "source"=""} ("error out") w202 w207 w214 w219 w225 w230 w237 w261 w278 w287 w299 w326 w331 w341 w345 w349 w353] -> w90
      tunnel: w85 -> [w122 w169 w177 w191 w196 w202 w207 w214 w220 w225 w231 w238 w262 w279 w288 w300 w326 w331 w341 w345 w349 w353]
      tunnel: [w125 w170 w175 w193 w199 w204 w208 w216 w222 w226 w233 w241 w276 w284 w290 w301 w327 w332 w342 w346 w350 w354] -> w89
      tunnel: [_ _ _ _ _ TRUE _ _ _ _ _ _ _ _ _ _ _ _ _ _ _ _] -> w88
      tunnel: [w121 w168 w174 w192 w197 w203 w206 w215 w218 w224 w232 w240 w267 w280 w289 w298 w325 w330 w340 w344 w348 w352] -> w87
      tunnel: w86 -> [w120 _ _ _ _ _ _ _ _ _ _ _ _ _ _ _ _ _ _ _ _ _]
      frame "", "Event Structure", "Idle" {
        n72 = event shown="[0] Timeout" {
          selector: _ -> [_ _ _ _ _]
          dyn-events: _ -> [_ _ _ _ _]
          timeout: w120 -> [_ _ _ _ _]
          tunnel: w126 -> [w130 w133 w139 w151 w167]
          tunnel: [w129 w132 w138 w150 w166] -> w125
          tunnel: w124 -> [w127 w135 w142 w155 w164]
          tunnel: [w128 w134 w140 w153 w165] -> w123
          tunnel: w122 -> [w128 w134 w141 w154 w165]
          tunnel: [w127 w135 w142 w155 w164] -> w121
          event Timeout {
            n73 = event-data() -> ()  [unwired: 1 in, 1 out]
            n74 = call <vilib>:"Add State(s) to Queue__jki_lib_state_machine.vi"("State(s) in (\"\")"=w130) -> ("States Out"=w129:string)  [unwired: 14 in]
          }
          event "stop": Value Change {
            n75 = event-data() -> ()  [unwired: 1 in, 6 out]
            n76 = call <vilib>:"Add State(s) to Queue__jki_lib_state_machine.vi"("State(s) in Front (\"\")"="Macro: Exit", "State(s) in (\"\")"=w133) -> ("States Out"=w132:string)  [unwired: 13 in]
          }
          event "GUIdevice 1": Value Change {
            n77 = event-data() -> ("NewVal"=w136:string)  [unwired: 1 in, 5 out]
            n78 = local write "GUIdevice 1"(w136) -> ()
            n79 = flat-sequence {
              tunnel: [w145] -> w140
              tunnel: w141 -> [w144]
              tunnel: w136 -> [w143]
              frame #0 {
                # "Set FP title as device name"
                n80 = control-ref of="This VI"() -> (w148:refnum<vi>)
                n81 = Concatenate Strings(w143, "_GUI ") -> (w147:string)
                n82 = property class="VI"(reference=w148, error in=w144, "Front Panel.Title"=w147) -> (error out=w145:errorcluster)  [unwired: 1 out]
              }
            }
            n83 = call <vilib>:"Add State(s) to Queue__jki_lib_state_machine.vi"("State(s) in Front (\"\")"="UI: Stop SuperGUI\nUI: Start SuperGUI", "State(s) in (\"\")"=w139) -> ("States Out"=w138:string)  [unwired: 13 in]
          }
          event "Select device": Value Change {
            n84 = event-data() -> ()  [unwired: 1 in, 6 out]
            n85 = local write "GUIdevice 1"("Select device") -> ()
            n86 = flat-sequence {
              tunnel: [w158] -> w153
              tunnel: w154 -> [w157]
              tunnel: "Select device" -> [w156]
              frame #0 {
                # "Set FP title as device name"
                n87 = control-ref of="This VI"() -> (w161:refnum<vi>)
                n88 = Concatenate Strings(w156, "_GUI ") -> (w160:string)
                n89 = property class="VI"(reference=w161, error in=w157, "Front Panel.Title"=w160) -> (error out=w158:errorcluster)  [unwired: 1 out]
              }
            }
            n90 = call <vilib>:"Add State(s) to Queue__jki_lib_state_machine.vi"("State(s) in Front (\"\")"="UI: Stop SuperGUI\nUI: Start SuperGUI", "State(s) in (\"\")"=w151) -> ("States Out"=w150:string)  [unwired: 13 in]
          }
          event Panel Close? {
            # "Discard the event because we'll close the front panel ourselves in Macro: Exit"
            # "Close Panel button (pressed) Event\n(this executes Macro: Exit to terminate the VI)"
            n91 = event-data() -> ()  [unwired: 1 in, 1 out]
            n92 = event-data("Discard?"=TRUE) -> ()  [unwired: 1 in, 1 out]
            n93 = call <vilib>:"Add State(s) to Queue__jki_lib_state_machine.vi"("State(s) in Front (\"\")"="Macro: Exit", "State(s) in (\"\")"=w167) -> ("States Out"=w166:string)  [unwired: 13 in]
          }
        }
      }
      frame "---------- Core ----------" {
        # "Do not put any code in this frame.\n(it is a separator no-op)"
        n94 = call <vilib>:"Add State(s) to Queue__jki_lib_state_machine.vi"("State(s) in (\"\")"=w171) -> ("States Out"=w170:string)  [unwired: 14 in]
      }
      frame Default {
        w181 = 42 items=["No error", "Argument error", "Memory is full", "Out of zone", "End of file", "File already open", "Generic file I/O error", "File not found", "File permission error", "Disk is full", "Duplicate path", "Too many files open", "System feature not enabled", "Resource file not found", "Cannot add resource", "Resource not found", "Image not found", "Image memory error", "Pen does not exist", "Config type invalid", "Config token not found", "Config parse error", "Config memory error", "Bad external code format", "Bad external code offset", "External code not present", "Null window", "Destroy window error", "Null menu", "Print aborted", "Bad print record", "Print driver error", "Windows error during printing", "Memory error during printing", "Print dialog error", "Generic print error", "Invalid device refnum", "Device not found", "Device parameter error", "Device unit error", "Cannot open device", "Device call aborted", "Generic error", "Cancelled by user", "Object ID too low", "Object ID too high", "Object not in heap", "Unknown heap", "Unknown object (invalid DefProc)", "Unknown object (DefProc not in table)", "Message out of range", "Invalid (null) method", "Unknown message", "Manager call not supported", "Bad address", "Network operation in progress", "Network operation timed out", "Connection is busy", "Network attribute not supported", "Network error", "Address in use", "System out of memory", "Connection aborted", "Connection refused", "Not connected", "Already connected", "Connection closed", "Initialization error (interapplication manager)", "Bad occurrence", "Wait on unbound occurrence handler", "Occurrence queue overflow", "Datalog type conflict", "Unused", "Unrecognized type (interapplication manager)", "Memory corrupt", "Failed to make temporary DLL", "Old CIN version", "Drag socket not found", "Failed to load drop-object", "Failed to register OLE object", "Failed to release OLE object", "Format specifier type mismatch", "Unknown format specifier", "Too few format specifiers", "Too many format specifiers", "Scan failed", "Newer CIN version", "Error converting to variant", "Runtime menu error", "Password tampered", "Variant attribute not found", "Incompatible variant data type", "Event data is not available", "Event Store is not present", "Occurrence is not found", "Event Queue is not created", "Event info is not available", "Refnum passed is NULL", "Error retrieving Class GUID", "Error retrieving CoClass GUID", "Error retrieving TypeLib GUID.", "Bad built application magic bytes.", "Specific driver is different from the specific driver associated with the Logical Name.", "There is no session opened to the class driver.", "Max Error", "MAX - Error with config objects", "MAX - Error loading configuration", "MAX - Group not supported"]
        # "Current State"
        # "Do not delete, rename, or modify this frame.\n(this is used to capture unhandled states and typos)"
        # "Handle mistyped state name (developer tool)"
        n95 = Format Into String(format string="Software Exception: Unhandled State \"%s\"." ("message"), error in=w177, w172) -> (resulting string=w180:string, error out=w179:errorcluster)  [unwired: 1 in]
        n96 = call <vilib>:"Error Cluster From Error Code.vi"("show call chain? (False)"=TRUE, "error in (no error)"=w179, "error message (\"\")"=w180, "error code (0)"=w181) -> ("error out"=w178:errorcluster)  [unwired: 5 in]
        n97 = call <vilib>:"Add State(s) to Queue__jki_lib_state_machine.vi"("State(s) in (\"\")"=w176) -> ("States Out"=w175:string)  [unwired: 14 in]
      }
      frame "Initialize Core Data" {
        # "Do not delete, rename, or modify this frame.\n(this is used to determine panel behavior on exit)"
        # "originally closed?"
        # "exe?"
        # "If panel starts closed or is an EXE, then close it when we exit"
        n98 = property class="VI"() -> ("Front Panel.Open"=w190:bool)  [unwired: 2 in, 2 out]
        n99 = property class="App"() -> ("App.Kind"=w189:T28)  [unwired: 2 in, 2 out]
        n100 = control-ref of="Current VI Reference"() -> (w183:refnum<vi>)
        n101 = Not(x=w190) -> (.not. x?=w187:bool)
        n102 = Equal?(x=w189, y=T28."Run Time System" ("Application:Kind")) -> (x = y?=w186:bool)
        n103 = Or(x=w187, y=w186) -> (x .or. y?=w184:bool)
        n104 = Bundle By Name(cluster=w185, "Core.Current VI Reference"=w183, "Core.Close Panel on Exit?"=w184) -> (w192:T31)
        n105 = call <vilib>:"Add State(s) to Queue__jki_lib_state_machine.vi"("State(s) in (\"\")"=w194) -> ("States Out"=w193:string)  [unwired: 14 in]
      }
      frame "Error Handler" {
        # "Unhandled Error -- Display it"
        # "Handle any errors here.\nYou can also output any states to clean-up after errors occur"
        # "Clear error"
        n106 = call <vilib>:"General Error Handler.vi"("error in (no error)"=w196) -> ()  [unwired: 10 in, 5 out]
        n107 = call <vilib>:"Add State(s) to Queue__jki_lib_state_machine.vi"("State(s) in Front (\"\")"="/* Post Error States", "State(s) in (\"\")"=w200) -> ("States Out"=w199:string)  [unwired: 13 in]
      }
      frame "Exit" {
        # "Do not put any code in this frame.\n(No errors that occur here will be handled.)"
        n108 = call <vilib>:"Add State(s) to Queue__jki_lib_state_machine.vi"("State(s) in (\"\")"=w205) -> ("States Out"=w204:string)  [unwired: 14 in]
      }
      frame "---------- Data ----------" {
        # "Do not put any code in this frame.\n(It is a separator no-op. You can make a copy of this frame to create a new Data frame)"
        n109 = call <vilib>:"Add State(s) to Queue__jki_lib_state_machine.vi"("State(s) in (\"\")"=w209) -> ("States Out"=w208:string)  [unwired: 14 in]
      }
      frame "Data: Initialize" {
        w210 = T32 {"STOP queue"=refnum, "SuperGUI ref"=refnum}  # SuperGUI
        w211 = T33 {"Current VI Reference"=refnum, "Close Panel on Exit?"=FALSE}  # Core
        w213 = TRUE  # Your Boolean data
        # "Initialize the shift-register data, here.\n(data names are defined by what you wire into the bundle function)"
        n110 = Bundle("Core"=w211, "Your Boolean data"=w213, "active cams"="active cams", "SuperGUI"=w210) -> (w215:T31)  [unwired: 1 in]
        n111 = call <vilib>:"Add State(s) to Queue__jki_lib_state_machine.vi"("State(s) in (\"\")"=w217) -> ("States Out"=w216:string)  [unwired: 14 in]
      }
      frame "Data: Cleanup" {
        # "Cleanup any data and references, here.\n(this is called automatically, by the Macro: Exit)"
        n112 = Unbundle By Name(w218) -> ("Core.Current VI Reference"=w221:refnum<vi>)
        n113 = Close Reference(reference=w221, error in (no error)=w220) -> (error out=w219:errorcluster)
        n114 = call <vilib>:"Add State(s) to Queue__jki_lib_state_machine.vi"("State(s) in (\"\")"=w223) -> ("States Out"=w222:string)  [unwired: 14 in]
      }
      frame "---------- UI ----------" {
        # "Do not put any code in this frame.\n(It is a separator no-op. You can make a copy of this frame to create a new UI frame)"
        n115 = call <vilib>:"Add State(s) to Queue__jki_lib_state_machine.vi"("State(s) in (\"\")"=w227) -> ("States Out"=w226:string)  [unwired: 14 in]
      }
      frame "UI: Initialize" {
        # "Initialize the User Interface, here.\n(this is called automatically, by the Macro: Init)"
        n116 = for {
          tunnel: string[] ["Point Grey Camera", "Manta Camera", "Photometrics Cam", "Basler Camera"] -> [w236] mode=indexing
          tunnel: [w235] -> w228 mode=concatenating
          n117 = call "getDevices.vi"("Device Class"=w236) -> ("All Devices"=w235:string[])
        }
        n118 = call <userlib>:"Fit VI window to Largest Dec__ogtk.vi"("error in (no error)"=w231) -> ("error out"=w230:errorcluster)  [unwired: 5 in, 1 out]
        n119 = property on="Select device" class="CmbBox"("Strings[]"=w228) -> ()  [unwired: 2 in, 2 out]
        n120 = call <vilib>:"Add State(s) to Queue__jki_lib_state_machine.vi"("State(s) in (\"\")"=w234) -> ("States Out"=w233:string)  [unwired: 14 in]
      }
      frame "UI: Get Device Name" {
        # "Initialize the User Interface, here.\n(this is called automatically, by the Macro: Init)"
        n121 = First Call?() -> (First Call?: T/F=w239:bool)
        n122 = case shown="True" w239 {
          tunnel: w238 -> [w243 w245]
          tunnel: [w243 w244] -> w237
          frame False {
          }
          frame True {
            n123 = disable-structure "Get Device name from control for vi mode\nand command line arg for exe" shown="RUN_TIME_ENGINE==True" {
              disable-tunnel: w245 -> [w246 w248]
              disable-tunnel: [w246 w247] -> w244
              frame condition #0 (active) {
              }
              frame condition #1 {
                n124 = control-ref of="This Application"() -> (w256:refnum<vi>)
                n125 = property class="App"(reference=w256) -> ("App.Args"=w255:string[])  [unwired: 1 in, 2 out]
                n126 = Index Array(array=w255, index #1=1 ("index")) -> (element #1=w249:string)  [unwired: 2 in, 2 out]
                n127 = Empty String/Path?(string/path=w249) -> (empty?=w253:bool)
                n128 = control-ref of="This VI"() -> (w252:refnum<vi>)
                n129 = case shown="False" w253 {
                  tunnel: w249 -> [w257 _]
                  frame False {
                    n130 = local write "GUIdevice 1"(w257) -> ()
                  }
                  frame True {
                  }
                }
                n131 = Concatenate Strings(w249, "_GUI ") -> (w251:string)
                n132 = property class="VI"(reference=w252, error in=w248, "Front Panel.Title"=w251) -> (error out=w247:errorcluster)  [unwired: 1 out]
              }
            }
          }
        }
        n133 = call <vilib>:"Add State(s) to Queue__jki_lib_state_machine.vi"("State(s) in (\"\")"=w242) -> ("States Out"=w241:string)  [unwired: 14 in]
      }
      frame "UI: Start SuperGUI" {
        # "create stop queue for supergui and its clones"
        # "x100 abort will be dependent on caller VI\nx80 abort will be independent of caller vi, this will abort vi when labview is closed."
        # "Start SuperGUI asynchronous way"
        n134 = vi-ref "GUI_Master_subvi_reentrant_queues.vi"() -> (w260:refnum<vi>)
        n135 = property class="VI"(reference=w260) -> ("Path"=w259:path)  [unwired: 1 in, 2 out]
        n136 = Create User Event(user event datatype=T29 {"EventEnum"=enum."new data", "Device name"="Device name"} ("New Event"), error in=w262) -> (user event=w263:refnum<user-event>, error out=w269:errorcluster)
        "tcp data event" <- w263
        n137 = control-ref of="This Application"() -> (w266:refnum<vi>)
        n138 = control-ref of="This VI"() -> (w265:refnum<vi>)
        n139 = Open VI Reference(type specifier VI Refnum (for type only)=refnum<vi> refnum, vi path=w259, options=256) -> (vi reference=w275:refnum<vi>, error out=w274:errorcluster)  [unwired: 3 in]
        n140 = register-events(w263) -> ()  [unwired: 2 in, 2 out]
        n141 = call "supergui create stop queue.vi"() -> ("STOP Queue out"=w271:refnum<queue>)  [unwired: 11 in]
        n142 = Current VI's Menubar() -> (w264:refnum<k9>)
        n143 = call-by-ref "Start Asynchronous Call"(reference=w275, error in=w274, "STOP Queue in"=w271, "This Application"=w266, 8:"error in (no error)"=w269, "tcp data event"=w263, "Caller menu reference"=w264, "Caller VI ref"=w265) -> (reference out=w258:refnum<vi>, error out=w261:errorcluster)  [unwired: 5 in, 1 out]
        n144 = Bundle By Name(cluster=w268, "SuperGUI.SuperGUI ref"=w258, "SuperGUI.STOP queue"=w271) -> (w267:T31)
        n145 = call <vilib>:"Add State(s) to Queue__jki_lib_state_machine.vi"("State(s) in (\"\")"=w277) -> ("States Out"=w276:string)  [unwired: 14 in]
      }
      frame "UI: Stop SuperGUI" {
        # "Stop Supergui Clone and wait until it exit properly"
        n146 = Unbundle By Name(w280) -> ("SuperGUI.SuperGUI ref"=w282:refnum<vi>, "SuperGUI.STOP queue"=w281:refnum<queue>)
        n147 = Release Queue(queue=w281, error in (no error)=w279) -> (error out=w283:errorcluster)  [unwired: 1 in, 2 out]
        n148 = call-by-ref "Wait On Asynchronous Call"(reference=w282, error in=w283) -> ("error out"=w278:errorcluster)  [unwired: 11 in, 2 out]
        n149 = call <vilib>:"Add State(s) to Queue__jki_lib_state_machine.vi"("State(s) in (\"\")"=w285) -> ("States Out"=w284:string)  [unwired: 14 in]
      }
      frame "UI: Cursor Set" {
        # "Argument"
        # "Set and Unset Cursor Busy.\n(Usage: \"UI: Cursor Set >> Busy|Idle\")"
        n150 = case shown="\"Idle\", Default" w286 {
          tunnel: w288 -> [w293 w295]
          tunnel: [w292 w294] -> w287
          frame "Idle", Default {
            n151 = call <vilib>:"Unset Busy.vi"("error in (no error)"=w293) -> ("error out"=w292:errorcluster)  [unwired: 10 in]
          }
          frame "Busy" {
            n152 = call <vilib>:"Set Busy.vi"("error in (no error)"=w295) -> ("error out"=w294:errorcluster)  [unwired: 9 in, 1 out]
          }
        }
        n153 = call <vilib>:"Add State(s) to Queue__jki_lib_state_machine.vi"("State(s) in (\"\")"=w291) -> ("States Out"=w290:string)  [unwired: 14 in]
      }
      frame "UI: Front Panel State" {
        # "Argument"
        # "Set Front Panel Open or Closed\n(Usage: \"UI: Front Panel State >> Open|Close\")"
        n154 = Unbundle By Name(w298) -> ("Core.Current VI Reference"=w297:refnum<vi>)
        n155 = case shown="\"Open\", Default" w296 {
          tunnel: w300 -> [w306 w319]
          tunnel: [w308 w320] -> w299
          tunnel: w297 -> [w307 w317]
          frame "Open", Default {
            n156 = property class="VI"(reference=w307, error in=w306) -> (reference out=w304:refnum<vi>, error out=w305:errorcluster, "Front Panel.Open"=w303:bool)
            n157 = case shown="False" w303 {
              tunnel: [w311 w314] -> w308
              tunnel: w305 -> [w310 w314]
              tunnel: w304 -> [w309 _]
              frame False {
                n158 = invoke class="VI" method="FP.Open"(reference=w309, error in=w310, "Activate"=TRUE, "State"=T30."Standard") -> (error out=w311:errorcluster)  [unwired: 1 in, 4 out]
              }
              frame True {
              }
            }
          }
          frame "Close" {
            n159 = property class="VI"(reference=w317, error in=w319) -> (reference out=w316:refnum<vi>, error out=w318:errorcluster, "Front Panel.Open"=w315:bool)
            n160 = case shown="True" w315 {
              tunnel: [w321 w324] -> w320
              tunnel: w318 -> [w321 w323]
              tunnel: w316 -> [_ w322]
              frame False {
              }
              frame True {
                n161 = invoke class="VI" method="FP.Close"(reference=w322, error in=w323) -> (error out=w324:errorcluster)  [unwired: 1 in, 2 out]
              }
            }
          }
        }
        n162 = call <vilib>:"Add State(s) to Queue__jki_lib_state_machine.vi"("State(s) in (\"\")"=w302) -> ("States Out"=w301:string)  [unwired: 14 in]
      }
      frame "---------- Macro ----------" {
        # "Do not put any code in this frame.\n(It is a separator no-op. You can make a copy of this frame to create a new Macro frame)"
        n163 = call <vilib>:"Add State(s) to Queue__jki_lib_state_machine.vi"("State(s) in (\"\")"=w328) -> ("States Out"=w327:string)  [unwired: 14 in]
      }
      frame "Macro: Initialize" {
        # "Initialization Macro\n(This is called once, when the VI starts)"
        n164 = call <vilib>:"Add State(s) to Queue__jki_lib_state_machine.vi"("State(s) in Front (\"\")"="Data: Initialize\nInitialize Core Data\nUI: Initialize\nUI: Get Device Name\nUI: Start SuperGUI\nUI: Front Panel State >> Open", "State(s) in (\"\")"=w333) -> ("States Out"=w332:string)  [unwired: 13 in]
      }
      frame "Macro: Exit" {
        # "Exit Macro\n(This is called once, when the VI exits)"
        n165 = Unbundle By Name(w340) -> ("Core.Close Panel on Exit?"=w339:bool)
        n166 = Select(t="UI: Front Panel State >> Close", s=w339, f="") -> (s? t:f=w336:string)
        n167 = call <vilib>:"Add State(s) to Queue__jki_lib_state_machine.vi"("State(s) in (\"\")"=w336, "State(s) at Back (\"\")"="Data: Cleanup\nExit") -> ("States Out"=w334:string)  [unwired: 13 in]
        n168 = call <vilib>:"Add State(s) to Queue__jki_lib_state_machine.vi"("State(s) in Front (\"\")"=w334, "State(s) in (\"\")"=w343) -> ("States Out"=w342:string)  [unwired: 13 in]
      }
      frame "---------- New Category ----------" {
        # "Template Separator\n(You can make a copy of, or modify, this frame)"
        n169 = call <vilib>:"Add State(s) to Queue__jki_lib_state_machine.vi"("State(s) in (\"\")"=w347) -> ("States Out"=w346:string)  [unwired: 14 in]
      }
      frame "New Category: 1" {
        # "Your code here.\n(You can make a copy of, or modify, this frame)"
        n170 = call <vilib>:"Add State(s) to Queue__jki_lib_state_machine.vi"("State(s) in (\"\")"=w351) -> ("States Out"=w350:string)  [unwired: 14 in]
      }
      frame "New Category: 2" {
        # "Your code here.\n(You can make a copy of, or modify, this frame)"
        n171 = call <vilib>:"Add State(s) to Queue__jki_lib_state_machine.vi"("State(s) in (\"\")"=w355) -> ("States Out"=w354:string)  [unwired: 14 in]
      }
    }
    n172 = for {
      tunnel: w84 -> [w111]
      tunnel: w83 -> [w115]
      tunnel: w81 -> [w112] mode=indexing
      tunnel: w80 -> [w108]
      (unwired) u32 16774656 ("Color")
      n173 = call-poly <userlib>:"Filter 1D Array__ogtk.vi"("items to filter"=w112, "array"=w115) -> ("filtered item indices"=w116:i32[])  [unwired: 4 in, 1 out]
      n174 = Index Array(array=w116) -> (element=w110:i32)  [unwired: 1 in]
      n175 = Index Array(array=w108, index=w110) -> (element=w109:T20)
      n176 = Unbundle By Name(w109) -> ("TargetSize.X::10"=w107:refnum<vi>, "TargetSize.Y::10"=w106:refnum<vi>)
      n177 = Index Array(array=w111, index=w110) -> (element=w114:T7)
      n178 = property class="DigNum (strict)"(reference=w107) -> ("Value"=w105:dbl)  [unwired: 1 in, 2 out]
      n179 = property class="DigNum (strict)"(reference=w106) -> ("Value"=w104:dbl)  [unwired: 1 in, 2 out]
      n180 = Unbundle By Name(w114) -> ("Target.X::10"=w118:refnum<vi>, "Target.Y::10"=w117:refnum<vi>)
      n181 = property class="DigNum (strict)"(reference=w117) -> ("Value"=w99:dbl)  [unwired: 1 in, 2 out]
      n182 = property class="DigNum (strict)"(reference=w118) -> ("Value"=w100:dbl)  [unwired: 1 in, 2 out]
      n183 = Bundle("Value"=w100, "Value"=w99) -> (w98:cluster{"Value":dbl, "Value":dbl})  [unwired: 1 in]
      n184 = Bundle("Value"=w105, "Value"=w104) -> (w97:cluster{"Value":dbl, "Value":dbl})  [unwired: 1 in]
      n185 = Bundle By Name(cluster=T26 {"Draw"=TRUE, "Target"={"x"=20.0, "y"=20.0}, "Size"={"x"=20.0, "y"=20.0}, "Angle"=1250067.0, "Color"=1250067, "Thickness"=5, "CrosshairLabel"=""} ("Crosshair"), "Draw"=TRUE, "Target"=w98, "Size"=w97, "Angle"=0.0, "Color"="Color") -> (w102:T26)
      n186 = call "draw crosshair imaq.vi"("Crosshair"=w102, "Bounding Rectangle"=T27 {"Left"=0, "Top"=0, "Right"=0, "Bottom"=0}, "image in"=w112) -> ("error out"=→"error out":errorcluster)  [unwired: 7 in, 1 out]
    }
  }
